vi "WPI_CounterStop.vi"(8 "error in (no error)":errorcluster, 11 "CounterDevRef in":T1) -> (0 "error out":errorcluster, 3 "CounterDevRef out":T1)   [LabVIEW 2017]
doc: "Stops the counter that you specify but does not reset the counter to zero. Use the Reset VI if you want to reset the counter without stopping the counter.\n\nThis software is licensed. Open the labview\\readme\\WPI Robotics Library Open Source License.txt file for more information."
uses:
  <vilib>/Rock Robotics/WPI/Counter/WPI_CounterDevRef.ctl
  <vilib>/Rock Robotics/SystemInterfaces/Counter/FPGA_CounterCtrSystemIndex.ctl
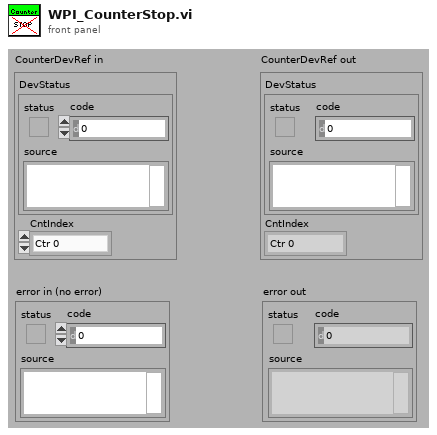
[diagram p1: front panel]
types:
  T1 = typedef "WPI_CounterDevRef.ctl" = cluster{"DevStatus":errorcluster, "CntIndex":T2}
  T2 = typedef "FPGA_CounterCtrSystemIndex.ctl" = enum8{"Ctr 0", "Ctr 1", "Ctr 2", "Ctr 3", "Ctr 4", "Ctr 5", "Ctr 6", "Ctr 7", "Invalid"}
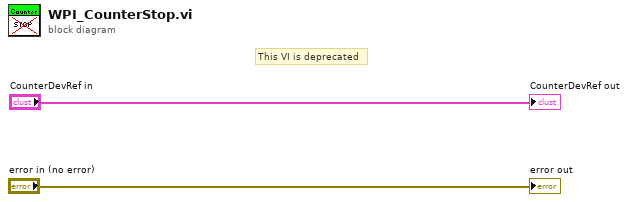
[diagram p0: block diagram]
diagram:
  # "This VI is deprecated"
  "CounterDevRef out" <- "CounterDevRef in"
  "error out" <- "error in (no error)"
